vi "Set Current.vi"(8 "error in":errorcluster, 10 "Current":dbl, 11 "Power Supply in":refnum<class "Power Supply.lvclass">) -> (0 "error out":errorcluster, 3 "Power Supply out":refnum<class "Power Supply.lvclass">)   [LabVIEW 2018, in "Power Supply.lvlib" / "Power Supply.lvclass"]
doc: "This VI updates the configuration for the output current and sends the updated settings to the power supply."
uses:
  Power Supply.lvclass
  Power Supply.lvclass/Power Supply.ctl
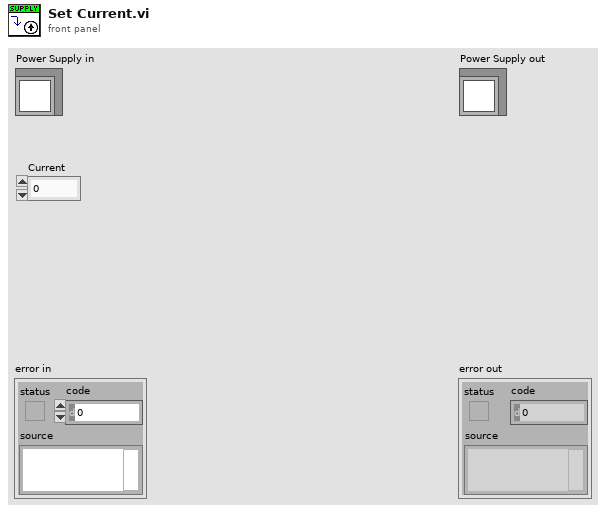
[diagram p1: front panel]
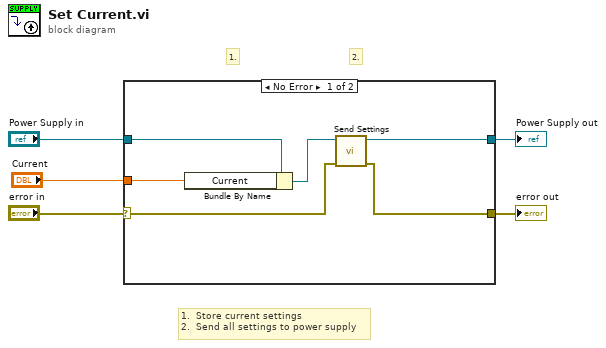
[diagram p0: block diagram]
diagram:
  # "1.  Store current settings\n2.  Send all settings to power supply"
  # "2."
  # "1."
  n1 = case shown="No Error" "error in" {
    selector: "error in" -> [w9 w13]
    tunnel: [w8 w13] -> w4
    tunnel: [w10 w12] -> w2
    tunnel: "Power Supply in" -> [w11 w12]
    tunnel: "Current" -> [w6 _]
    frame No Error {
      n2 = Bundle By Name(cluster=w11, "Current"=w6) -> (w7:refnum<class "Power Supply.lvclass">)
      n3 = call-dynamic "Send Settings.vi"("error in (no error)"=w9, "Power Supply in"=w7) -> ("error out"=w8:errorcluster, "Power Supply out"=w10:refnum<class "Power Supply.lvclass">)  [unwired: 8 in]
    }
    frame Error {
    }
  }
  "error out" <- w4
  "Power Supply out" <- w2
